vi "HasMLERangeChanged1.vi"(0 "WFGraph Refnum":refnum<vi>) -> (1 "Selection Changed":bool, 2 "output range":cluster{"x0":dbl, "x1":dbl})   [LabVIEW 2009]
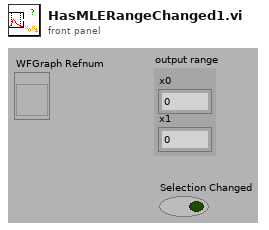
[diagram p1: front panel]
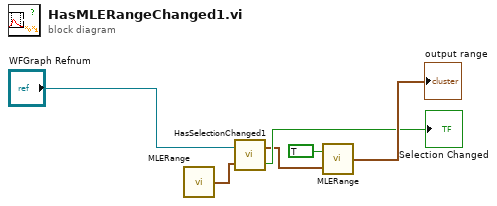
[diagram p0: block diagram]
diagram:
  n1 = call "MLERange.vi"() -> ("output range"=w1:cluster{"x0":dbl, "x1":dbl})  [unwired: 2 in]
  n2 = call "HasSelectionChanged1.vi"("input range"=w1, "WFGraph Refnum"="WFGraph Refnum") -> ("Selection Changed"=→"Selection Changed":bool, "output range"=w2:cluster{"x0":dbl, "x1":dbl})
  n3 = call "MLERange.vi"("input range"=w2, "set"=TRUE) -> ("output range"=→"output range":cluster{"x0":dbl, "x1":dbl})
